vi "Set Config Analog Out.vi"(0 "hdwf":i32, 1 "vAmplitude":dbl=1.0, 2 "degPhase":dbl, 5 "idxChannel":i32, 7 "node":T2, 9 "hzFrequency":dbl, 11 "error in (no error)":errorcluster, 12 "vOffset":dbl, 13 "func":T1 items=["DC"=0, "Sine"=1, "Square"=2, "Triangle"=3, "RampUp"=4, "RampDown"=5, "Noise"=6, "Custom"=30, "Play"=31]) -> (4 "hdwf out":i32, 15 "error out":errorcluster)   [LabVIEW 2014, in "AnalogDiscSDKLv.lvlib"]
doc: "extern \"C\" __declspec(dllexport) int SetConfig_AnalogOut(\n HDWF hdwf, \n int idxChannel,\n AnalogOutNode node,\n double hzFrequency, \n double vAmplitude, \n double vOffset,\n double degPhase,\n FUNC func\n );"
uses:
  <instrlib>/AnalogDiscSDKLv/AnalogDiscSDKLv.lvlib
  <instrlib>/AnalogDiscSDKLv/VIs/DWF_Node.ctl
  <instrlib>/AnalogDiscSDKLv/VIs/DWF_Function.ctl
  <instrlib>/AnalogDiscSDKLv/AnalogDiscSDKLv.dll
panel:
  out "Numeric":i32
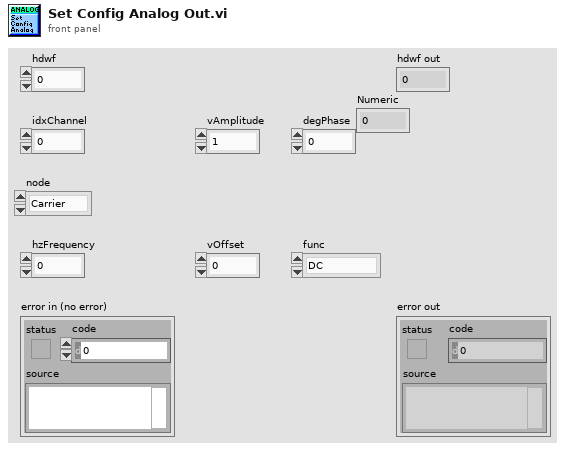
[diagram p1: front panel]
types:
  T1 = typedef "AnalogDiscSDKLv.lvlib/DWF_Function.ctl" = u8
  T2 = typedef "AnalogDiscSDKLv.lvlib/DWF_Node.ctl" = enum16{"Carrier", "FM", "AM"}
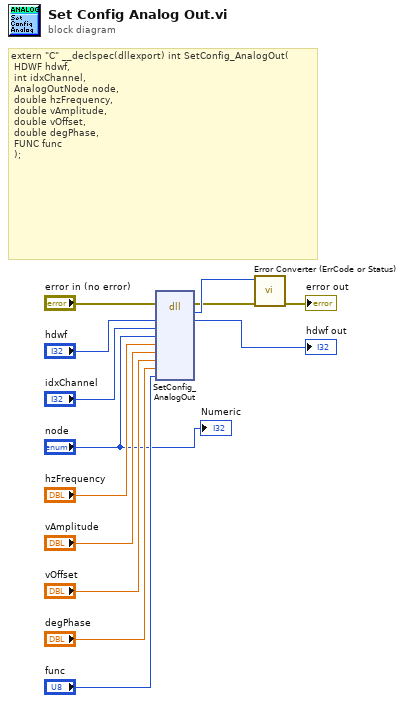
[diagram p0: block diagram]
diagram:
  # "extern \"C\" __declspec(dllexport) int SetConfig_AnalogOut(\n\tHDWF hdwf, \n\tint idxChannel,\n\tAnalogOutNode node,\n\tdouble hzFrequency, \n\tdouble vAmplitude, \n\tdouble vOffset,\n\tdouble degPhase,\n\tFUNC func\n\t);"
  n1 = dll-call lib="C:/Program Files (x86)/National Instruments/LabVIEW 2014/instr.lib/AnalogDiscSDKLv/AnalogDiscSDKLv.*" fn="SetConfig_AnalogOut"(error in="error in (no error)", "hdwf"="hdwf", "idxChannel"="idxChannel", "node"="node", "hzFrequency"="hzFrequency", "vAmplitude"="vAmplitude", "vOffset"="vOffset", "degPhase"="degPhase", "func"="func") -> (error out=w3:errorcluster, "return type"=w4:i32, "hdwf"=→"hdwf out":i32)  [unwired: 9 in, 1 out]
  n2 = call <instrlib>:"Error Converter (ErrCode or Status).vi"("error in (no error)"=w3, "error code"=w4) -> ("error out"=→"error out":errorcluster)  [unwired: 9 in]
  "Numeric" <- "node"
